vi "MALT Set Several.vi"(7 "MALT CardType":T1=enum."MALT132", 8 "error in":errorcluster, 9 "State":bool, 10 "State Map":u8[](array[numeric]) format="%02x", 11 "Address":i32) -> (0 "error out":errorcluster)   [LabVIEW 2018]
uses:
  Types/MALT CardTypes.ctl
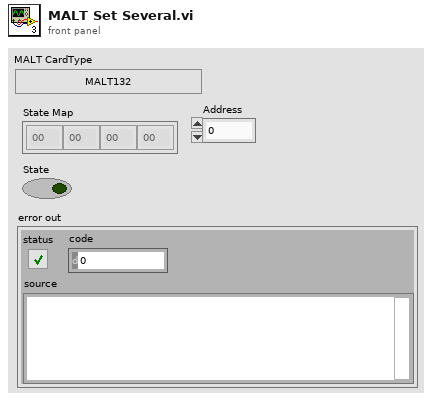
[diagram p1: front panel]
types:
  T1 = typedef "MALT CardTypes.ctl" = enum32{"-", "YAV90832", "YAV904X8", "MALT132", "YAV91616", "YAV90PIN", "YAV90096", "YAV90HVT", "YAV90CLR", "YAV90128", "YAV90PNE", "YAVCANCON", "YAV91775", "YAV90XXX", "YAV90MMU", "H730050", "H710060", "H710061", "YAV90304", "MMI", "YAV90060", "YAV90MUX", "YAV90059", "Not Defined"}
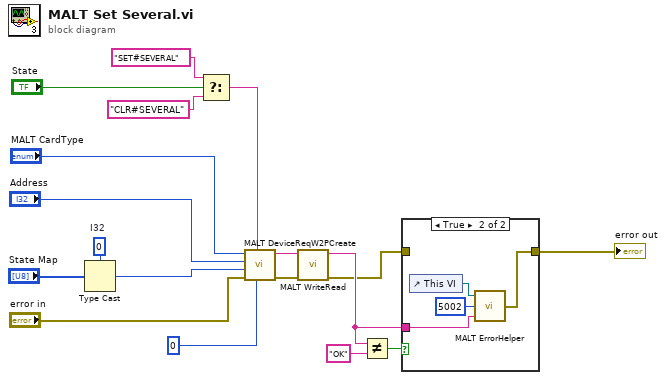
[diagram p0: block diagram]
diagram:
  w3 = 0  # I32
  n1 = Type Cast(type=w3, x="State Map") -> (*(type *) &x=w2:i32)
  n2 = Select(t="SET#SEVERAL" ("cmd"), s="State", f="CLR#SEVERAL" ("cmd")) -> (s? t:f=w8:string)
  n3 = call "MALT DeviceReqW2PCreate.vi"("Param2"=0, "Cmd"=w8, "error in"="error in", "Param1"=w2, "Address"="Address", "CardType"="MALT CardType") -> ("error out"=w17:errorcluster, "Request"=w18:string)  [unwired: 4 in]
  n4 = call "MALT WriteRead.vi"("error in"=w17, "Request"=w18) -> ("error out"=w9:errorcluster, "Response"=w11:string)  [unwired: 8 in]
  n5 = Not Equal?(x=w11, y="OK") -> (x != y?=w12:bool)
  n6 = case shown="True" w12 {
    tunnel: w11 -> [_ w21]
    tunnel: [w19 w20] -> w10
    tunnel: w9 -> [w19 _]
    frame False {
    }
    frame True {
      n7 = control-ref of="This VI"() -> (w23:refnum<vi>)
      n8 = call "MALT ErrorHelper.vi"("Message"=w21, "Code"=5002, "This VI"=w23) -> ("error out"=w20:errorcluster)
    }
  }
  "error out" <- w10
